vi "save and close project.vi"(8 "error in (no error)":errorcluster, 11 "Project in":refnum<vi>) -> (0 "error out":errorcluster)   [LabVIEW 2024]
doc: "saves and closes the project reference"
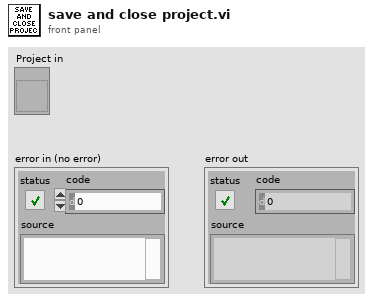
[diagram p1: front panel]
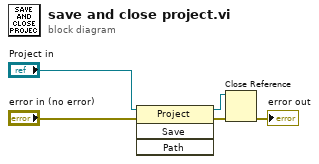
[diagram p0: block diagram]
diagram:
  n1 = invoke class="Project" method="Save"(reference="Project in", error in="error in (no error)") -> (reference out=w3:refnum<vi>, error out=w2:errorcluster)  [unwired: 2 in, 2 out]
  n2 = Close Reference(reference=w3, error in (no error)=w2) -> (error out=→"error out":errorcluster)
